vi "FPGA Image Recording (Host).vi"() -> ()   [LabVIEW 2013]
doc: "This is the host VI for the 10-Tap 8-Bit Camera with DRAM example. This example demonstrates how to acquire images from a 10-tap, 8-bit, extended configuration, Camera Link camera and display the images on the host. This example supports area scan and line scan cameras for both continuous and finite acquisitions.\n\nThis example also demonstrates the use of DRAM as a frame buffer for very high speed acquisitions. Data packing and flow-control are also employed to maximize use of the available DRAM and FIFOs in terms of both memory space and performance.\n\nAdditionally, the example demonstrates the serial server, which allows third-party camera configuration utilities to communicate with the camera using the Camera Link serial interface while this VI is running."
uses:
  <vilib>/userdefined/High Color/nirio_resource_hc.ctl
  Network Stream/Network Stream Module Enum.ctl
  <vilib>/rvi/interface/common/niFpgaWaitOnOcc.vi
  <vilib>/FPGAPlugInAG/PCIe-1473R/niLvFpga_Open_PCIe-1473R.vi
  <vilib>/rvi/interface/common/dynamic/niFpgaDynamicAddResources.vi
  <vilib>/FPGAPlugInAG/Dynamic/niLvFpga_Reset_Dynamic.vi
  <vilib>/Utility/error.llb/Error Cluster From Error Code.vi
  <vilib>/rvi/errors/niLvFpgaAdjustHostInterfaceError.vi
  <vilib>/FPGAPlugInAG/Dynamic/niLvFpga_Run_Dynamic.vi
  <vilib>/FPGAPlugInAG/Dynamic/niLvFpga_Close_Dynamic.vi
  <vilib>/rvi/interface/nirviOpenFPGA/nirviOpenFPGA.xnode
  FPGA Bitfiles/10-Tap8-bitwith_DRAM.lvbitx
  <vilib>/rvi/interface/nirviMethod/nirviMethod.xnode
  <vilib>/rvi/interface/nirviReadWriteControl/nirviReadWriteControl.xnode
  <vilib>/rvi/interface/nirviCloseFPGA/nirviCloseFPGA.xnode
  <vilib>/rvi/interface/Simulation/niFpgaSimulationCallBeginRW.vi
  <vilib>/rvi/errors/niLvFpgaMergeErrorWithErrorCode.vi
  NiFpgaLv.dll
  <vilib>/FPGAPlugInAG/Dynamic/niLvFpga_ConfigureFifo_Dynamic.vi
  <vilib>/FPGAPlugInAG/Dynamic/niLvFpga_StartFifo_Dynamic.vi
  <vilib>/FPGAPlugInAG/Dynamic/niLvFpga_ReadFifo_Dynamic.vi
panel:
  out "# of lost frames":u32
  in  "Record?":bool
  in  "DMA Buffer Size\n(In Images)":u32=64 caption="DMA Buffer Size"
  in  "Signal Mapping":T1(ring)=enum."Basler 10-tap"
  out "Acq In Progress":bool=TRUE
  in  "Line Scan":bool
  in  "Frames To Acquire":u32 caption="Frames To Acquire\n(0 = infinite)"
  in  "Cancel":bool
  out "Acq'd Frame Width":u32=2040
  in  "Stopped":bool=TRUE
  in  "RIO Device":T2="RIO0"
  out "DMA Write Timeout":bool
  in  "Start Serial Server":bool=TRUE
  out "Frames Acq'd":u32=49
  out "Acq'd Frame Height":u32=1088
  out "Image":T3(plugin-control)
  in  "Acquire":bool
  in  "Stop":bool
  in  "Image Height":u32=1088 max=65535
  in  "Image Width":u32=2040 max=65535 step=40
  out "Initialized":bool
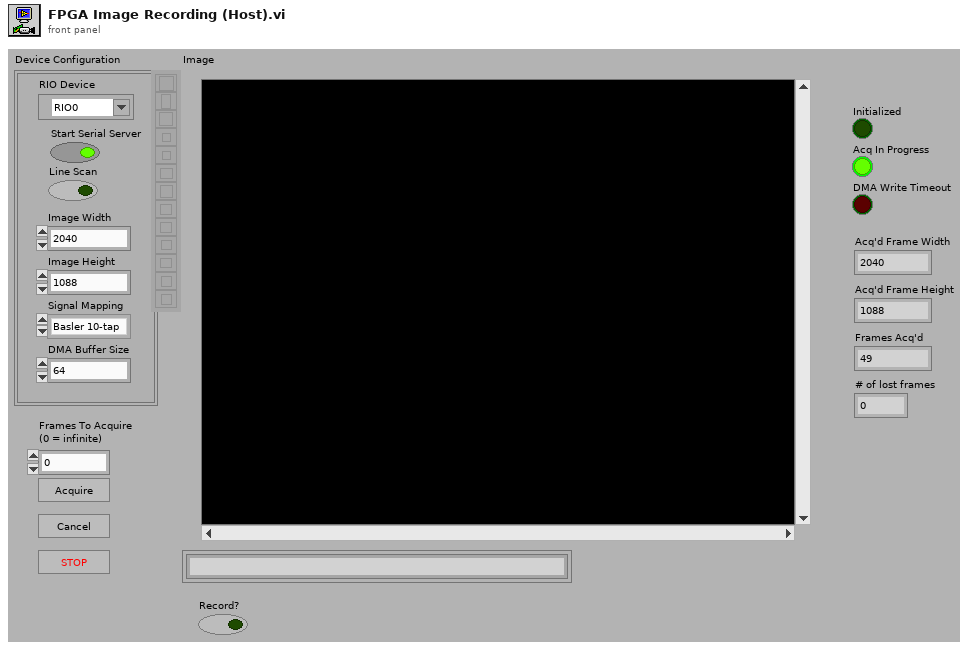
[diagram p1: front panel]
types:
  T1 = enum8{"Standard", "Basler 10-tap", "Vosskühler 10-tap"}
  T2 = typedef "nirio_resource_hc.ctl" = tag
  T3 = typedef "IMAQ Image.ctl" = refnum<image>
  T4 = typedef "Image Type" = u32
  T5 = typedef "Network Stream Module Enum.ctl" = enum16{"Initialize", "Write", "Close"}
  T6 = enum16{"big-endian, network order", "native, host order", "little-endian"}
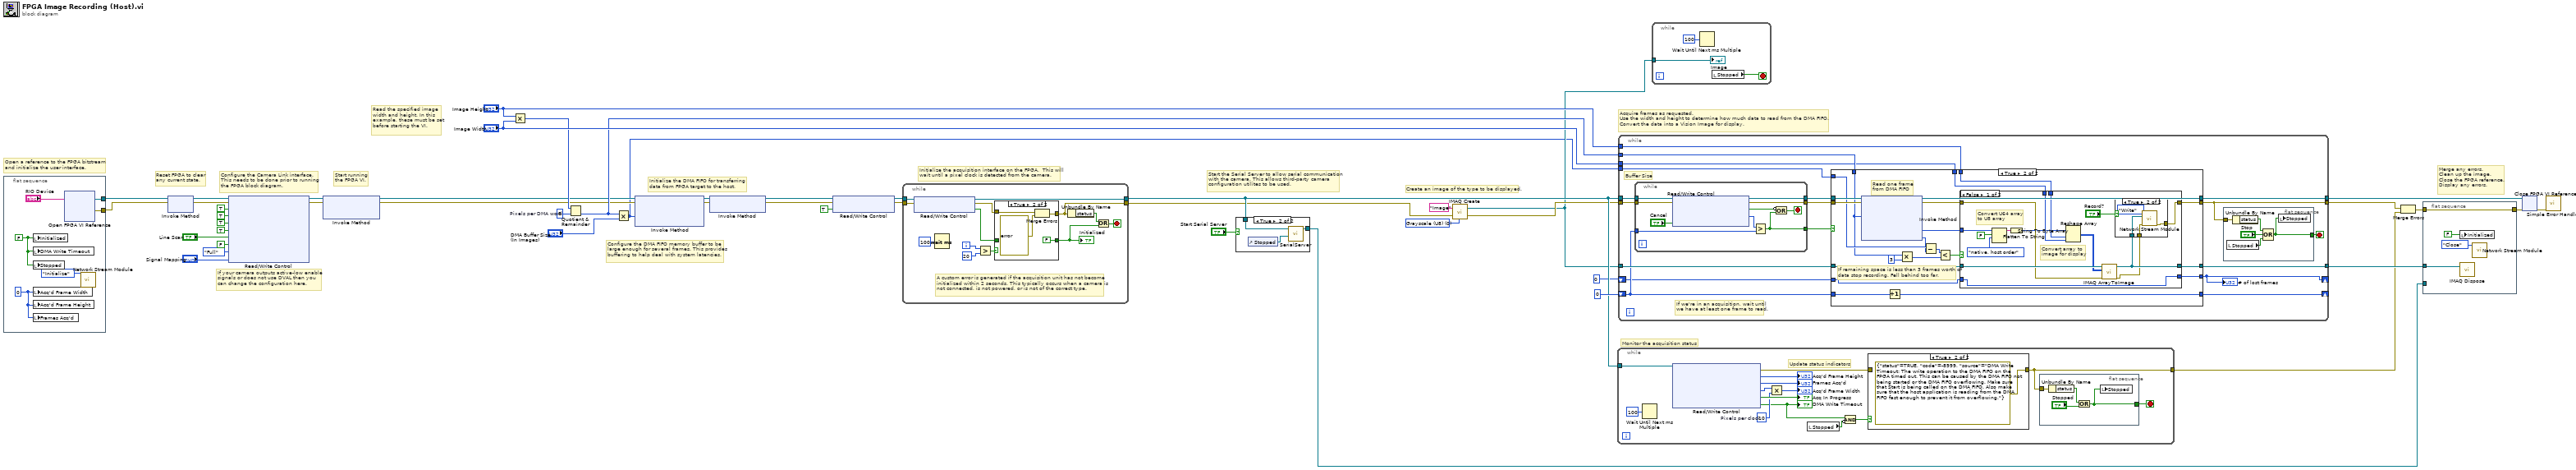
[diagram p0: block diagram]
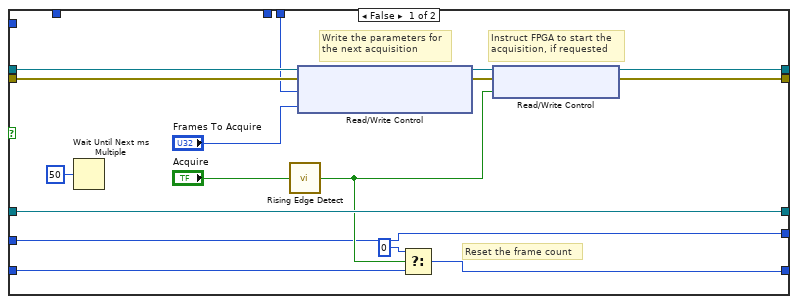
[diagram p4: hidden frame]
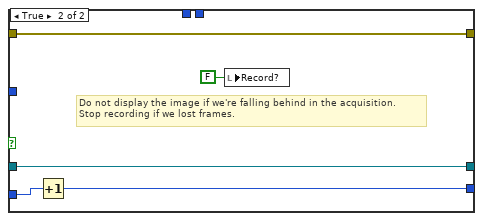
[diagram p6: hidden frame]
diagram:
  w9 = u32 8  # Pixels per DMA word
  w43 = T4 0 items=["Grayscale (U8)", "Grayscale (I16)", "Grayscale (SGL)", "Complex (CSG)", "RGB (U32)", "HSL (U32)", "RGB (U64)", "Grayscale (U16)"] ("Image Type")
  # "If your camera outputs active-low enable\nsignals or does not use DVAL then you \ncan change the configuration here."
  # "Configure the DMA FIFO memory buffer to be\nlarge enough for several frames. This provides\nbuffering to help deal with system latencies."
  # "Start running\nthe FPGA VI."
  # "Reset FPGA to clear\nany current state."
  # "Read the specified image\nwidth and height. In this\nexample, these must be set\nbefore starting the VI."
  # "Merge any errors.\nClean up the image.\nClose the FPGA reference.\nDisplay any errors."
  # "Acquire frames as requested.\nUse the width and height to determine how much data to read from the DMA FIFO.\nConvert the data into a Vision Image for display."
  # "Monitor the acquisition status"
  # "Start the Serial Server to allow serial communication\nwith the camera. This allows third-party camera\nconfiguration utilites to be used."
  # "Create an image of the type to be displayed."
  # "Initialize the acquisition interface on the FPGA.  This will\nwait until a pixel clock is detected from the camera."
  # "Initialize the DMA FIFO for transferring\ndata from FPGA target to the host."
  # "Configure the Camera Link interface.\nThis needs to be done prior to running\nthe FPGA block diagram."
  # "Open a reference to the FPGA bitstream\nand initialize the user interface."
  n1 = flat-sequence {
    tunnel: [w50] -> w34
    tunnel: [w49] -> w47
    frame #0 {
      w53 = u32 0 ("Num Lines Acq'd")
      w52 = FALSE ("stop")
      n2 = local write "Initialized"(w52) -> ()
      n3 = local write "DMA Write Timeout"(w52) -> ()
      n4 = local write "Stopped"(w52) -> ()
      n5 = local write "Acq'd Frame Width"(w53) -> ()
      n6 = local write "Acq'd Frame Height"(w53) -> ()
      n7 = local write "Frames Acq'd"(w53) -> ()
      n8 = xnode "Open FPGA VI Reference"("resource name"="RIO Device") -> ("FPGA VI Reference Out"=w50:refnum<k20>, "error out"=w49:errorcluster)  [unwired: 1 in]
      n9 = call "Network Stream Module.vi"("Operation"=Network_Stream_Module_Enum."Initialize") -> ()  [unwired: 10 in, 1 out]
    }
  }
  n10 = xnode "Invoke Method"("FPGA VI Reference In"=w34, "error in"=w47) -> ("FPGA VI Reference Out"=w23:refnum<k20>, "error out"=w26:errorcluster)
  n11 = xnode "Read/Write Control"("FPGA VI Reference In"=w23, "error in"=w26, "CL Config.FVAL Active High"=TRUE ("IO Module Config.CL FVAL Active High"), "CL Config.LVAL Active High"=TRUE ("IO Module Config.CL LVAL Active High"), "CL Config.DVAL Active High"=TRUE ("IO Module Config.CL DVAL Active High"), "CL Config.Spare Active High"=TRUE ("IO Module Config.CL Spare Active High"), "CL Config.Line Scan"="Line Scan", "Acq Control.Ignore DVAL"=FALSE ("CL Config.Line Scan"), "CL Config.Configuration"=enum8{"Base", "Medium", "Full"}."Full", "CL Config.Signal Mapping"="Signal Mapping") -> ("FPGA VI Reference Out"=w27:refnum<k20>, "error out"=w25:errorcluster)
  n12 = xnode "Invoke Method"("FPGA VI Reference In"=w27, "error in"=w25) -> ("FPGA VI Reference Out"=w6:refnum<k20>, "error out"=w5:errorcluster)  [unwired: 1 in]
  n13 = Multiply(x="Image Height", y="Image Width") -> (x*y=w8:u32)
  n14 = Quotient & Remainder(x=w8, y=w9) -> (floor(x/y)=w7:u32)  [unwired: 1 out]
  n15 = Multiply(x=w7, y="DMA Buffer Size\n(In Images)") -> (x*y=w1:u32)
  n16 = xnode "Invoke Method"("FPGA VI Reference In"=w6, "error in"=w5, "Requested Depth"=w1) -> ("FPGA VI Reference Out"=w33:refnum<k20>, "error out"=w32:errorcluster)  [unwired: 1 out]
  n17 = xnode "Invoke Method"("FPGA VI Reference In"=w33, "error in"=w32) -> ("FPGA VI Reference Out"=w18:refnum<k20>, "error out"=w31:errorcluster)
  n18 = xnode "Read/Write Control"("FPGA VI Reference In"=w18, "error in"=w31, "Acq Control.Initialize"=TRUE ("Arm Acquisition")) -> ("FPGA VI Reference Out"=w46:refnum<k20>, "error out"=w45:errorcluster)
  n19 = while {
    tunnel: w46 -> [w61]
    tunnel: w45 -> [w60]
    tunnel: [w59] -> w15
    tunnel: [w63] -> w14
    i -> [w55]
    stop <- w66 stop-if-true
    # "A custom error is generated if the acquisition unit has not become\ninitialized within 2 seconds. This typically occurs when a camera is\nnot connected, is not powered, or is not of the correct type."
    n20 = xnode "Read/Write Control"("FPGA VI Reference In"=w61, "error in"=w60) -> ("FPGA VI Reference Out"=w59:refnum<k20>, "error out"=w58:errorcluster, "Acq Status.Initialized"=w57:bool)
    n21 = Wait (ms)(milliseconds to wait=u32 100) -> ()  [unwired: 1 out]
    n22 = Greater?(x=w55, y=20) -> (0:w56:bool)
    n23 = case shown="True" w56 {
      tunnel: [w68 FALSE] -> w62
      tunnel: w57 -> [w68 _]
      tunnel: w58 -> [w67 w70]
      tunnel: [w67 w72] -> w63
      frame False {
      }
      frame True {
        n24 = Merge Errors(w70, errorcluster {"status"=TRUE, "code"=-8999, "source"="Acquisition Initialization: This error typically occurs when a camera is not properly connected, is not powered, or is not of the correct type."} ("error in")) -> (w72:errorcluster)
      }
    }
    "Initialized" <- w62
    n25 = Unbundle By Name(w63) -> ("status"=w65:bool)
    n26 = Or(x=w65, y=w62) -> (x .or. y?=w66:bool)
  }
  n27 = case shown="True" "Start Serial Server" {
    tunnel: [_ w73] -> w35
    tunnel: w15 -> [_ w74]
    frame False {
    }
    frame True {
      n28 = control-ref of="Stopped"() -> (w75:refnum<vi>)
      n29 = call "SerialServer.vi"("Stop Refnum"=w75, "FPGA VI Reference In"=w74) -> ("FPGA VI Reference Out"=w73:refnum<k20>)  [unwired: 5 in]
    }
  }
  n30 = call "IMAQ Create"("Image Name"="Image", "Image Type"=w43, "error in (no error)"=w14) -> ("New Image"=w2:T3, "error out"=w4:errorcluster)  [unwired: 2 in]
  n31 = while {
    tunnel: w15 -> [w86]
    tunnel: [w89] -> w28
    stop <- w88 stop-if-true
    w79 = u32 10  # Pixels per clock
    # "Update status indicators"
    n32 = Wait Until Next ms Multiple(millisecond multiple=u32 100) -> ()  [unwired: 1 out]
    n33 = xnode "Read/Write Control"("FPGA VI Reference In"=w86) -> ("error out"=w85:errorcluster, "Acq Status.Lines Per Frame"=→"Acq'd Frame Height":u32, "Acq Status.Frames Acq'd"=→"Frames Acq'd":u32, "Acq Status.Clocks Per Line"=w80:u32, "Acq Status.Acq In Progress"=→"Acq In Progress":bool, "Acq Status.DMA Write Timeout"=w77:bool)  [unwired: 1 in, 1 out]
    "DMA Write Timeout" <- w77
    n34 = Multiply(x=w80, y=w79) -> (x*y=→"Acq'd Frame Width":u32)
    n35 = local read "Stopped"() -> (w76:bool)
    n36 = Compound Arithmetic op=AND(w77, invert w76) -> (w78:bool)
    n37 = case shown="True" w78 {
      tunnel: w85 -> [w94 _]
      tunnel: [w94 errorcluster {"status"=TRUE, "code"=-8999, "source"="DMA Write Timeout: The write operation to the DMA FIFO on the FPGA timed out. This can be caused by the DMA FIFO not being started or the DMA FIFO overflowing. Make sure that Start is being called on the DMA FIFO. Also make sure that the host application is reading from the DMA FIFO fast enough to prevent it from overflowing."} ("error out")] -> w89
      frame False {
      }
      frame True {
      }
    }
    n38 = flat-sequence {
      tunnel: w89 -> [w93]
      tunnel: [w91] -> w88
      frame #0 {
        n39 = Unbundle By Name(w93) -> ("status"=w92:bool)
        n40 = Or(x=w92, y="Stopped") -> (x .or. y?=w91:bool)
        n41 = local write "Stopped"(w91) -> ()
      }
    }
  }
  n42 = while {
    tunnel: w15 -> [w105]
    tunnel: w4 -> [w104]
    tunnel: w7 -> [w113]
    tunnel: "Image Height" -> [w112]
    tunnel: "Image Width" -> [w111]
    tunnel: w2 -> [w110]
    tunnel: [w108] -> w29
    tunnel: [w109] -> w42
    tunnel: [w106] -> w37
    shift-right: [w100] -> _
    shift-left: u32 0 -> [w99]
    shift-right: [w98] -> _
    shift-left: u32 0 -> [w97]
    tunnel: w1 -> [w96]
    stop <- w107 stop-if-true
    # "Buffer Size"
    # "If we're in an acquisition, wait until\nwe have at least one frame to read."
    n43 = while {
      tunnel: w105 -> [w120]
      tunnel: w104 -> [w119]
      tunnel: [w117] -> w103
      tunnel: [w118] -> w102
      tunnel: w99 -> [w123]
      tunnel: [w121] -> w101
      stop <- w122 stop-if-true
      n44 = xnode "Read/Write Control"("FPGA VI Reference In"=w120, "error in"=w119, "Acq Control.Cancel Acq"="Cancel") -> ("FPGA VI Reference Out"=w118:refnum<k20>, "error out"=w117:errorcluster, "Acq Status.Acq In Progress"=w116:bool, "Acq Status.Frames Acq'd"=w115:u32)
      n45 = Greater?(x=w115, y=w123) -> (0:w121:bool)
      n46 = Compound Arithmetic op=OR(invert w116, w121) -> (w122:bool)
    }
    n47 = case shown="True" w101 {
      tunnel: w102 -> [w140 w158]
      tunnel: w103 -> [w139 w157]
      tunnel: w113 -> [_ w148]
      tunnel: w112 -> [w133 w165]
      tunnel: w111 -> [_ w164]
      tunnel: w110 -> [w144 w163]
      tunnel: [w135 w161] -> w108
      tunnel: [w138 w160] -> w109
      tunnel: [w144 w159] -> w106
      tunnel: w99 -> [w141 w156]
      tunnel: [w143 w155] -> w100
      tunnel: [w129 w152] -> w98
      tunnel: w97 -> [w129 w151]
      tunnel: w96 -> [_ w150]
      frame False {
        # "Reset the frame count"
        # "Instruct FPGA to start the\nacquisition, if requested"
        # "Write the parameters for\nthe next acquisition"
        n48 = Wait Until Next ms Multiple(millisecond multiple=u32 50) -> ()  [unwired: 1 out]
        n49 = call "Rising Edge Detect.vi"("Input"="Acquire") -> ("Pulse"=w130:bool)  [unwired: 4 in]
        n50 = xnode "Read/Write Control"("FPGA VI Reference In"=w140, "error in"=w139, "Acq Control.Line Scan Height"=w133, "Acq Control.Frames To Acq"="Frames To Acquire") -> ("FPGA VI Reference Out"=w137:refnum<k20>, "error out"=w136:errorcluster)
        n51 = Select(t=u32 0, s=w130, f=w141) -> (s? t:f=w143:u32)
        n52 = xnode "Read/Write Control"("FPGA VI Reference In"=w137, "error in"=w136, "Acq Control.Acquire"=w130) -> ("FPGA VI Reference Out"=w138:refnum<k20>, "error out"=w135:errorcluster)
      }
      frame True {
        # "If remaining space is less than 3 frames worth of data stop recording. Fell behind too far."
        # "Read one frame\nfrom DMA FIFO"
        n53 = xnode "Invoke Method"("FPGA VI Reference In"=w158, "error in"=w157, "Number of Elements"=w148) -> ("FPGA VI Reference Out"=w160:refnum<k20>, "error out"=w162:errorcluster, "Data"=w154:u64[], "Elements Remaining"=w149:u32)  [unwired: 1 in]
        n54 = Increment(x=w156) -> (x+1=w155:u32)
        n55 = Multiply(x=w148, y=u32 3) -> (x*y=w146:u32)
        n56 = Subtract(x=w150, y=w149) -> (x-y=w145:u32)
        n57 = Less?(x=w145, y=w146) -> (x < y?=w153:bool)
        n58 = case shown="False" w153 {
          tunnel: w165 -> [w180 _]
          tunnel: w164 -> [w179 _]
          tunnel: w163 -> [w178 w190]
          tunnel: w162 -> [w177 w189]
          tunnel: [w166 w189] -> w161
          tunnel: [w170 w190] -> w159
          tunnel: w154 -> [w174 _]
          tunnel: [w168 w188] -> w152
          tunnel: w151 -> [w168 w187]
          frame False {
            # "Convert U64 array\nto U8 array"
            # "Convert array to\nimage for display"
            n59 = Flatten To String(anything=w174, prepend array or string size? (T)=FALSE, byte order (0:big-endian, network order)=T6."native, host order") -> (data string=w172:string)  [unwired: 1 in, 2 out]
            n60 = String To Byte Array(string=w172) -> (unsigned byte array=w171:u8[])
            n61 = Reshape Array(w171, w180, w179) -> (w176:u8[][])
            n62 = call "IMAQ ArrayToImage"("error in (no error)"=w177, "Image Pixels (U8)"=w176, "Image"=w178) -> ("error out"=w167:errorcluster, "Image Out"=w170:T3)  [unwired: 7 in]
            n63 = case shown="True" "Record?" {
              tunnel: w170 -> [_ w182]
              tunnel: w167 -> [w181 w184]
              tunnel: [w181 w183] -> w166
              frame False {
              }
              frame True {
                n64 = call "Network Stream Module.vi"("error in (no error)"=w184, "Image In"=w182, "Operation"=Network_Stream_Module_Enum."Write") -> ("error out"=w183:errorcluster)  [unwired: 8 in]
              }
            }
          }
          frame True {
            # "Do not display the image if we're falling behind in the acquisition.\nStop recording if we lost frames."
            n65 = Increment(x=w187) -> (x+1=w188:u32)
            n66 = local write "Record?"(FALSE ("Record?")) -> ()
          }
        }
      }
    }
    "# of lost frames" <- w98
    n67 = flat-sequence {
      tunnel: w108 -> [w126]
      tunnel: [w125] -> w107
      frame #0 {
        n68 = local read "Stopped"() -> (w124:bool)
        n69 = Unbundle By Name(w126) -> ("status"=w127:bool)
        n70 = Compound Arithmetic op=OR(w127, "Stop", w124) -> (w125:bool)
        n71 = local write "Stopped"(w125) -> ()
      }
    }
  }
  n72 = while {
    tunnel: w2 -> [w193]
    stop <- w191 stop-if-true
    n73 = Wait Until Next ms Multiple(millisecond multiple=u32 100) -> ()  [unwired: 1 out]
    n74 = local read "Stopped"() -> (w191:bool)
    "Image" <- w193
  }
  n75 = Merge Errors(w29, w28) -> (w30:errorcluster)
  n76 = flat-sequence {
    tunnel: w30 -> [w196]
    tunnel: [w196] -> w39
    tunnel: w37 -> [w197]
    tunnel: w35 -> [_]
    frame #0 {
      n77 = local write "Initialized"(FALSE ("Module Enabled")) -> ()
      n78 = call "IMAQ Dispose"("Image"=w197) -> ()  [unwired: 5 in, 1 out]
      n79 = call "Network Stream Module.vi"("Operation"=Network_Stream_Module_Enum."Close") -> ()  [unwired: 10 in, 1 out]
    }
  }
  n80 = xnode "Close FPGA VI Reference"("FPGA VI Reference In"=w42, "error in"=w39) -> ("error out"=w36:errorcluster)
  n81 = call <vilib>:"Simple Error Handler.vi"("error in (no error)"=w36) -> ()  [unwired: 4 in, 5 out]
